vi "Organize PTR Results.vi"(7 "Check Array Order?":bool=TRUE, 8 "error in (no error)":errorcluster, 10 "Part Count":u16, 11 "PTRs W/Limits":refnum<class "PTR.lvclass">[](array[class])) -> (0 "error out":errorcluster, 3 "Sorted PTR":refnum<class "PTR.lvclass">[][](array[class]))   [LabVIEW 2018, in "STDF File Parser.lvclass"]
uses:
  STDF File Parser.lvclass
  <userlib>/STDF/PTR/PTR.lvclass
  <vilib>/Utility/error.llb/Error Cluster From Error Code.vi
  <vilib>/ErrorRing/Error Ring.xnode
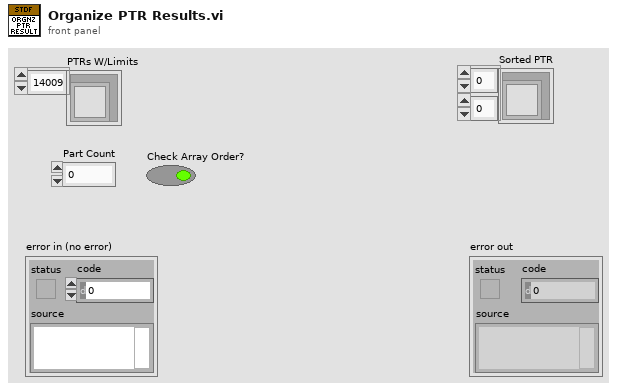
[diagram p1: front panel]
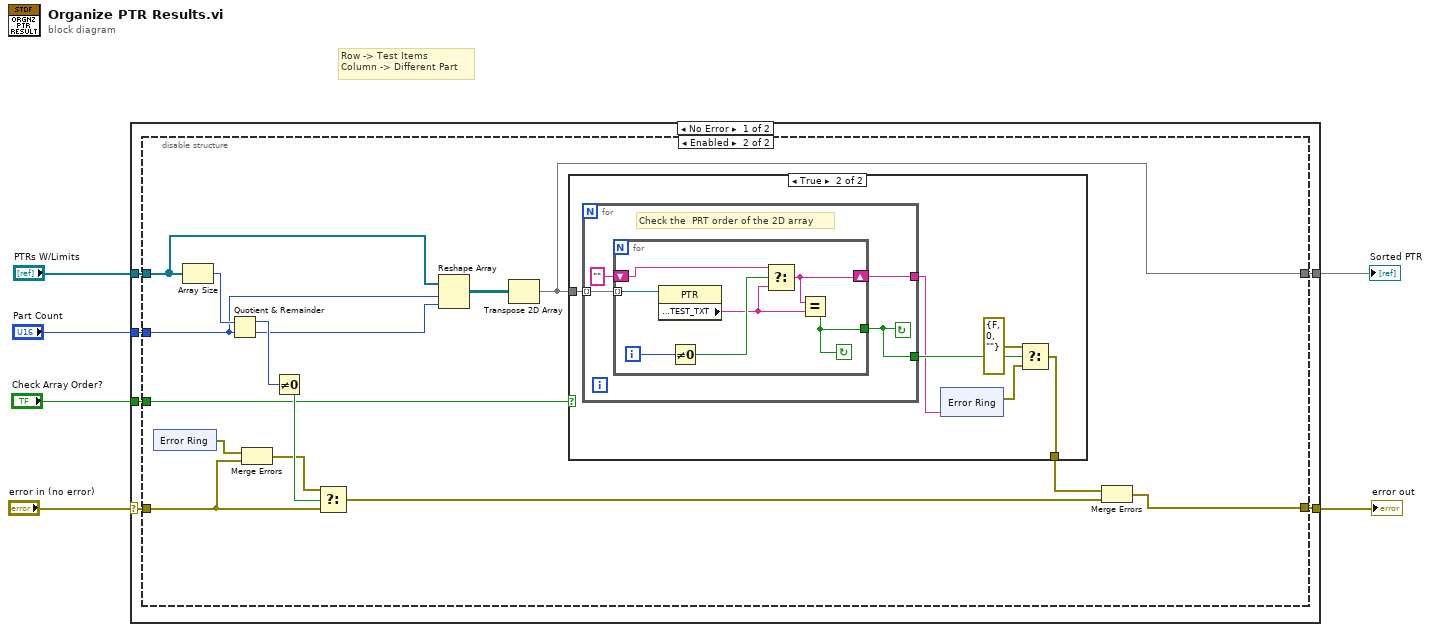
[diagram p0: block diagram]
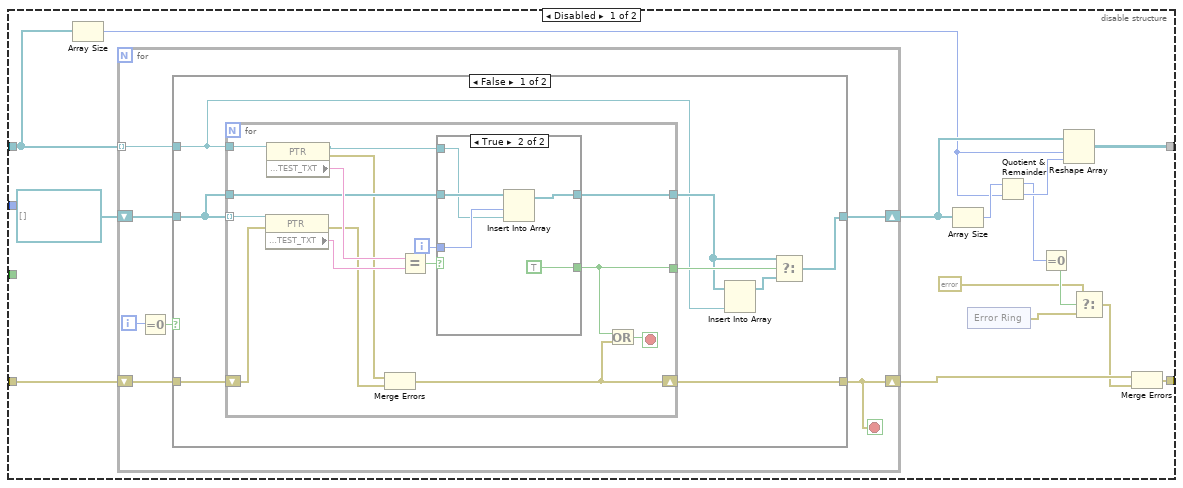
[diagram p2: hidden frame]
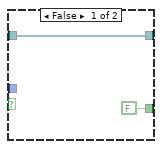
[diagram p3: hidden frame]
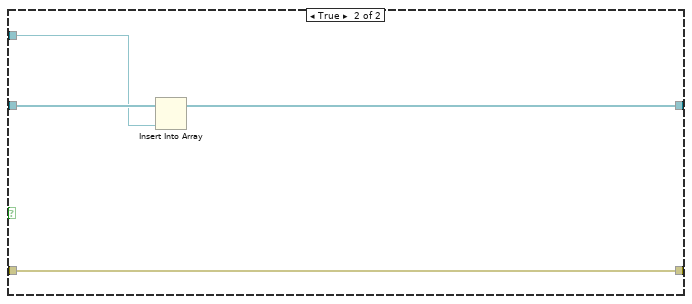
[diagram p4: hidden frame]
diagram:
  # "Row -> Test Items\nColumn -> Different Part"
  n1 = case shown="No Error" "error in (no error)" {
    selector: "error in (no error)" -> [w12 w118]
    tunnel: [w9 w118] -> w5
    tunnel: "PTRs W/Limits" -> [w11 _]
    tunnel: [w10 _] -> w3
    tunnel: "Part Count" -> [w8 _]
    tunnel: "Check Array Order?" -> [w7 _]
    frame No Error {
      n2 = disable-structure shown="Enabled" {
        disable-tunnel: w12 -> [w27 w83]
        disable-tunnel: w11 -> [w25 w82]
        disable-tunnel: [w20 w75] -> w10
        disable-tunnel: [w15 w76] -> w9
        disable-tunnel: w8 -> [_ w81]
        disable-tunnel: w7 -> [_ w74]
        frame Disabled {
          n3 = Array Size(array=w25) -> (size(s)=w22:i32)
          n4 = for {
            tunnel: w25 -> [w36] mode=indexing
            shift-right: [w33] -> w14
            shift-left: w27 -> [w34]
            shift-right: [w35] -> w23
            shift-left: refnum<class "PTR.lvclass">[] [] -> [w37]
            i -> [w39]
            stop <- w33 stop-if-true
            n5 = Equal To 0?(x=w39) -> (x = 0?=w38:bool)
            n6 = case shown="False" w38 {
              tunnel: w37 -> [w47 w73]
              tunnel: w36 -> [w42 w72]
              tunnel: [w44 w71] -> w35
              tunnel: w34 -> [w46 w70]
              tunnel: [w40 w70] -> w33
              frame False {
                n7 = for {
                  tunnel: w42 -> [w61]
                  tunnel: w47 -> [w62] mode=indexing
                  tunnel: w47 -> [w56]
                  tunnel: [w54] -> w43
                  tunnel: [w49] -> w45
                  shift-right: [w48] -> w40
                  shift-left: w46 -> [w53]
                  i -> [w55]
                  stop <- w50 stop-if-true
                  n8 = property class="PTR"(reference=w62, error in=w53) -> (error out=w51:errorcluster, "Accessors:TEST_TXT"=w59:string)  [unwired: 1 out]
                  n9 = property class="PTR"(reference=w61) -> (reference out=w57:refnum<class "PTR.lvclass">, error out=w52:errorcluster, "Accessors:TEST_TXT"=w60:string)  [unwired: 1 in]
                  n10 = Merge Errors(w52, w51) -> (w48:errorcluster)
                  n11 = Equal?(x=w60, y=w59) -> (x = y?=w58:bool)
                  n12 = case shown="True" w58 {
                    tunnel: w57 -> [_ w67]
                    tunnel: w56 -> [w64 w69]
                    tunnel: w55 -> [_ w68]
                    tunnel: [w64 w66] -> w54
                    tunnel: [FALSE TRUE] -> w49
                    frame False {
                    }
                    frame True {
                      n13 = Insert Into Array(array=w69, index=w68, new element=w67) -> (w66:refnum<class "PTR.lvclass">[])
                    }
                  }
                  n14 = Or(x=w49, y=w48) -> (x .or. y?=w50:bool)
                }
                n15 = Insert Into Array(array=w43, new element=w42) -> (w41:refnum<class "PTR.lvclass">[])  [unwired: 1 in]
                n16 = Select(t=w43, s=w45, f=w41) -> (s? t:f=w44:refnum<class "PTR.lvclass">[])
              }
              frame True {
                n17 = Insert Into Array(array=w73, new element=w72) -> (w71:refnum<class "PTR.lvclass">[])  [unwired: 1 in]
              }
            }
          }
          n18 = Array Size(array=w23) -> (size(s)=w24:i32)
          n19 = xnode "Error Ring"() -> ("error out"=w17:errorcluster)
          n20 = Quotient & Remainder(x=w24, y=w22) -> (x-y*floor(x/y)=w19:i32, floor(x/y)=w21:i32)
          n21 = Equal To 0?(x=w19) -> (x = 0?=w18:bool)
          n22 = Reshape Array(w23, w22, w21) -> (w20:refnum<class "PTR.lvclass">[][])
          n23 = Select(t=errorcluster {"status"=FALSE, "code"=0, "source"=""}, s=w18, f=w17) -> (s? t:f=w13:errorcluster)
          n24 = Merge Errors(w14, w13) -> (w15:errorcluster)
        }
        frame Enabled {
          n25 = xnode "Error Ring"() -> ("error out"=w87:errorcluster)
          n26 = Array Size(array=w82) -> (size(s)=w88:i32)
          n27 = Quotient & Remainder(x=w88, y=w81) -> (x-y*floor(x/y)=w85:i32, floor(x/y)=w80:i32)
          n28 = Merge Errors(w87, w83) -> (w84:errorcluster)
          n29 = Not Equal To 0?(x=w85) -> (x != 0?=w86:bool)
          n30 = Select(t=w84, s=w86, f=w83) -> (s? t:f=w78:errorcluster)
          n31 = Reshape Array(w82, w81, w80) -> (w79:refnum<class "PTR.lvclass">[][])
          n32 = Transpose 2D Array(2D array=w79) -> (transposed array=w75:refnum<class "PTR.lvclass">[][])
          n33 = case shown="True" w74 {
            tunnel: [_ w90] -> w77
            tunnel: w75 -> [_ w89]
            frame False {
            }
            frame True {
              n34 = for {
                tunnel: w89 -> [w105] mode=indexing
                tunnel: [w103] -> w92
                tunnel: [w102] -> w94
                stop <- w102 continue-if-true
                # "Check the  PRT order of the 2D array"
                n35 = for {
                  tunnel: w105 -> [w112] mode=indexing
                  shift-right: [w108] -> w103
                  shift-left: "" ("Accessors:TEST_TXT") -> [w109]
                  tunnel: [w106] -> w102
                  i -> [w111]
                  stop <- w106 continue-if-true
                  n36 = property class="PTR"(reference=w112) -> ("Accessors:TEST_TXT"=w107:string)  [unwired: 1 in, 2 out]
                  n37 = Not Equal To 0?(x=w111) -> (x != 0?=w110:bool)
                  n38 = Select(t=w109, s=w110, f=w107) -> (s? t:f=w108:string)
                  n39 = Equal?(x=w108, y=w107) -> (x = y?=w106:bool)
                }
              }
              n40 = xnode "Error Ring"("parameter 0"=w92) -> ("error out"=w93:errorcluster)
              n41 = Select(t=errorcluster {"status"=FALSE, "code"=0, "source"=""}, s=w94, f=w93) -> (s? t:f=w90:errorcluster)
            }
          }
          n42 = Merge Errors(w77, w78) -> (w76:errorcluster)
        }
      }
    }
    frame Error {
    }
  }
  "error out" <- w5
  "Sorted PTR" <- w3
